vi "Misc.vi"   [LabVIEW 2018]
uses:
  <vilib>/Rock Robotics/WPI/DriverStation/WPI_DriverStationRobotMode2.ctl
  <vilib>/Rock Robotics/Network Tables/NT Read Boolean.vi
  SubSystems/Drive Train/Drive Train Global.vi
  <vilib>/Rock Robotics/Network Tables/NT Read String.vi
  Robot Global Data.vi
  SubSystems/HAB Climber/HAB Climber Global.vi
  <vilib>/Rock Robotics/Network Tables/NT Write Boolean.vi
  SubSystems/Lift/Lift Global.vi
  SubSystems/Cargo Intake/Cargo Intake Global.vi
  SubSystems/Hatch Panel Intake/Hatch Panel Intake Global.vi
  <vilib>/Rock Robotics/Network Tables/NT Write Numeric Array.vi
  <vilib>/Rock Robotics/Network Tables/NT Write Number.vi
  SubSystems/Controllers/Driver Controller/Driver Controller Global.vi
  SubSystems/Controllers/Manipulator Controlller/Manipulator Controller Global.vi
types:
  T1 = typedef "WPI_DriverStationRobotMode2.ctl" = enum16{"Autonomous Disabled", "Autonomous Enabled", "Teleop Disabled", "Teleop Enabled", "Disconnected", "Finish", "Test Disabled", "Test Enabled", "Emergency Stopped"}
  T2 = typedef "WPI_CompressorDevRef.ctl" = cluster{"DevStatus":errorcluster, "Pneumatics Control Module":u8}
  T3 = cluster{"FrontLeft":dbl, "FrontRight":dbl, "BackLeft":dbl, "BackRight":dbl}
  T4 = cluster{"Rollover":dbl, "Yaw":dbl, "Cont Yaw":dbl}
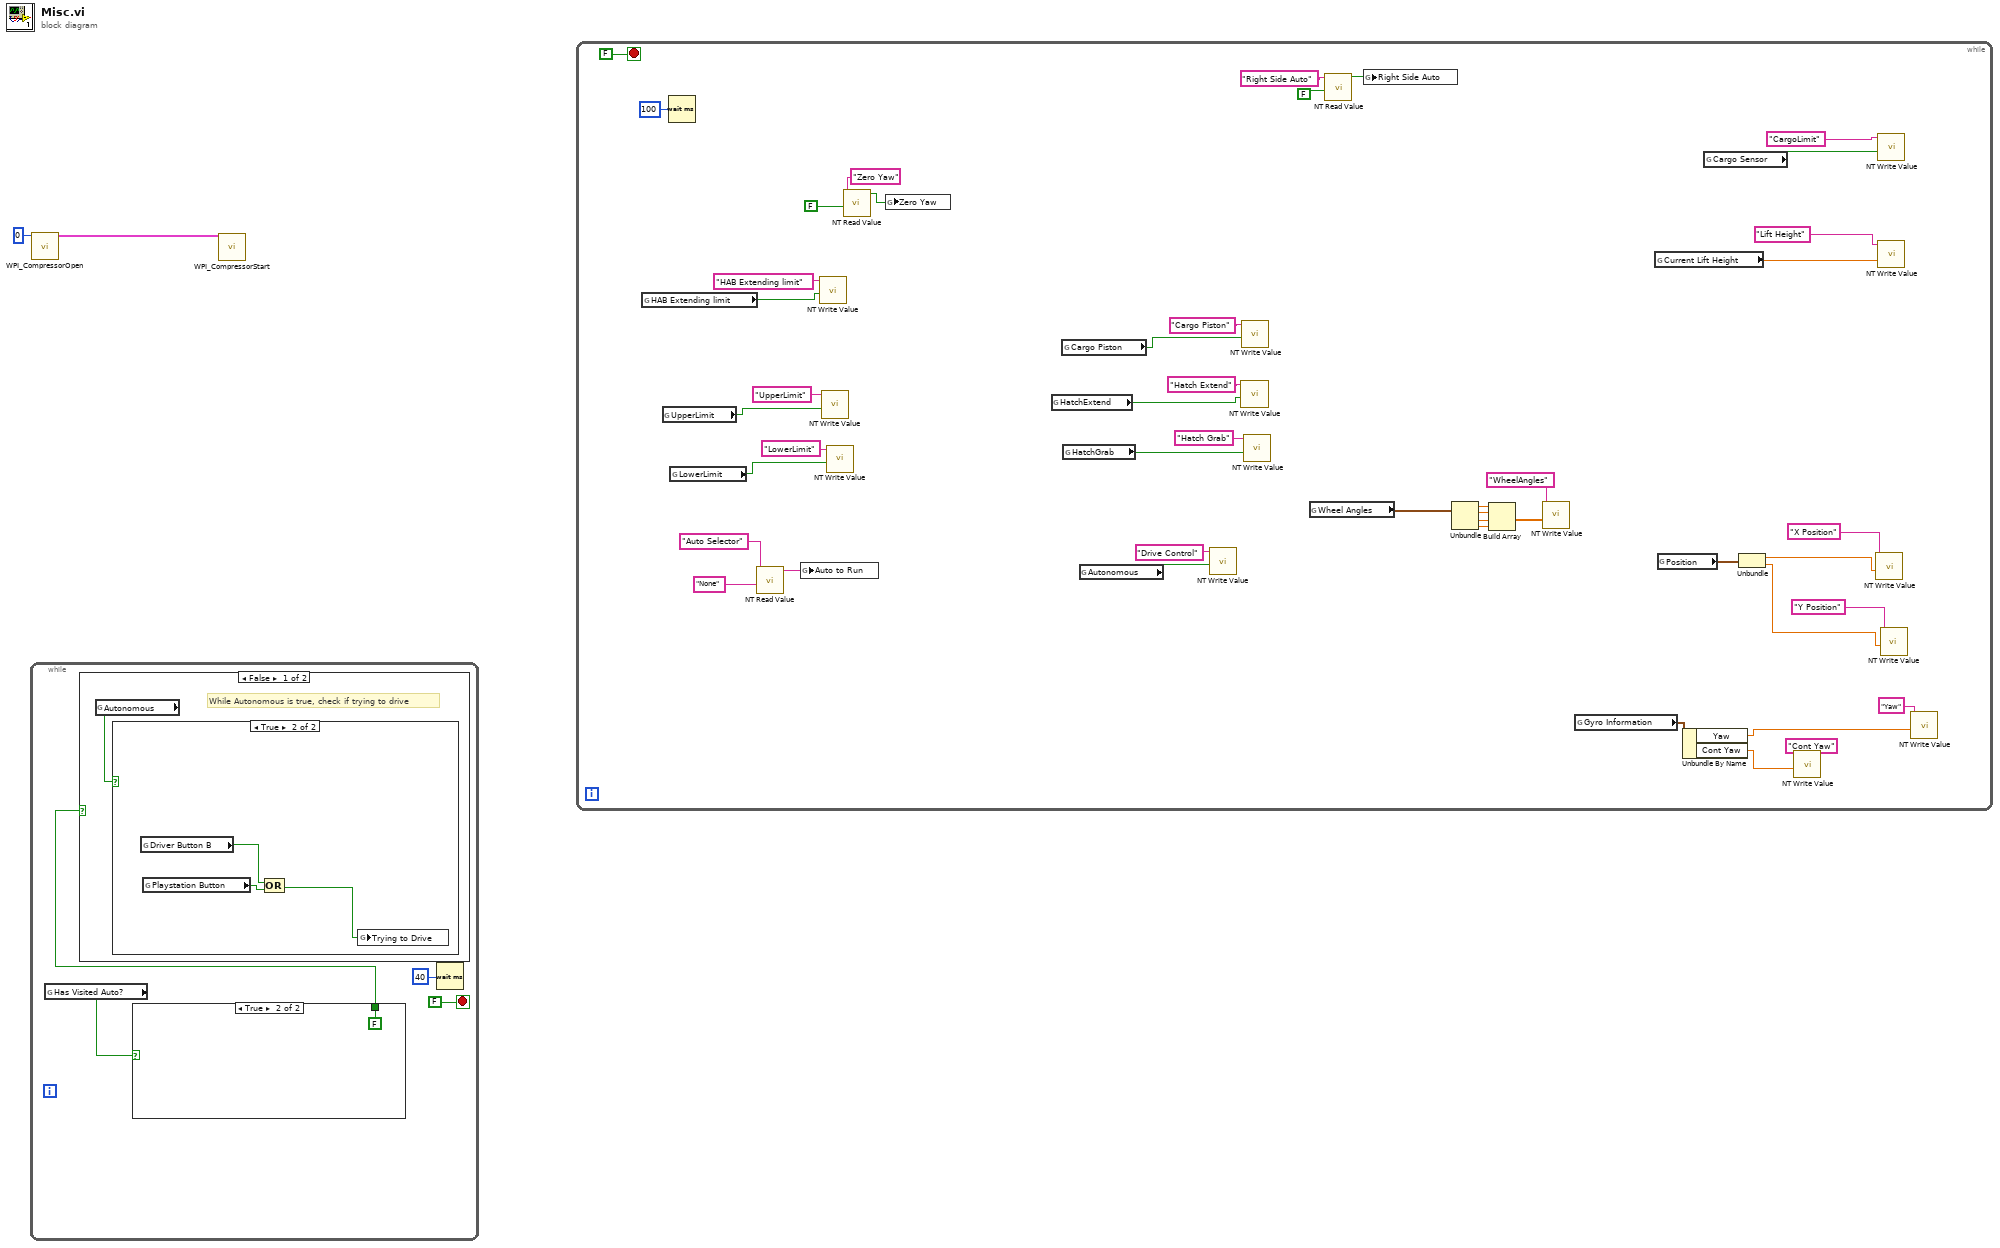
[diagram p0: block diagram]
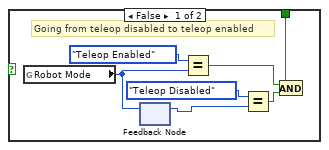
[diagram p2: hidden frame]
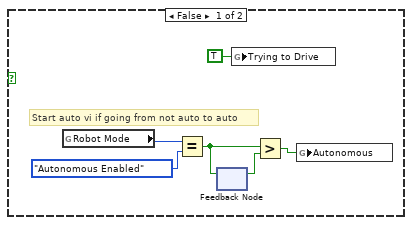
[diagram p3: hidden frame]
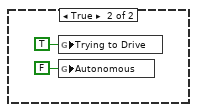
[diagram p4: hidden frame]
diagram:
  n1 = while {
    stop <- FALSE stop-if-true
    n2 = global read "Robot Global Data.vi" "Has Visited Auto?"() -> (w3:bool)
    n3 = case shown="True" w3 {
      tunnel: [w7 FALSE] -> w4
      frame False {
        # "Going from teleop disabled to teleop enabled"
        n4 = global read "Robot Global Data.vi" "Robot Mode"() -> (w13:T1)
        n5 = feedback #1() -> (w10:T1)  [unwired: 1 in]
        n6 = feedback-in #1(w13) -> ()
        n7 = Equal?(x=WPI_DriverStationRobotMode2."Teleop Enabled" ("y"), y=w13) -> (x = y?=w8:bool)
        n8 = Equal?(x=WPI_DriverStationRobotMode2."Teleop Disabled" ("y"), y=w10) -> (x = y?=w9:bool)
        n9 = And(x=w8, y=w9) -> (x .and. y?=w7:bool)
      }
      frame True {
      }
    }
    n10 = case shown="False" w4 {
      frame False {
        # "While Autonomous is true, check if trying to drive"
        n11 = global read "Robot Global Data.vi" "Autonomous"() -> (w15:bool)
        n12 = case shown="True" w15 {
          frame False {
            # "Start auto vi if going from not auto to auto"
            n13 = global read "Robot Global Data.vi" "Robot Mode"() -> (w17:T1)
            n14 = Equal?(x=w17, y=WPI_DriverStationRobotMode2."Autonomous Enabled") -> (x = y?=w18:bool)
            n15 = feedback #2() -> (w19:bool)  [unwired: 1 in]
            n16 = feedback-in #2(w18) -> ()
            n17 = global write "Robot Global Data.vi" "Trying to Drive"(TRUE ("Trying to Drive")) -> ()
            n18 = Greater?(x=w18, y=w19) -> (0:w20:bool)
            n19 = global write "Robot Global Data.vi" "Autonomous"(w20) -> ()
          }
          frame True {
            n20 = global read "Driver Controller Global.vi" "Driver Button B"() -> (w23:bool)
            n21 = global read "Manipulator Controller Global.vi" "Playstation Button"() -> (w22:bool)
            n22 = Compound Arithmetic op=OR(w23, w22) -> (w24:bool)
            n23 = global write "Robot Global Data.vi" "Trying to Drive"(w24) -> ()
          }
        }
      }
      frame True {
        n24 = global write "Robot Global Data.vi" "Trying to Drive"(TRUE ("Trying to Drive")) -> ()
        n25 = global write "Robot Global Data.vi" "Autonomous"(FALSE ("Autonomous")) -> ()
      }
    }
    n26 = Wait (ms)(milliseconds to wait=u32 40) -> ()  [unwired: 1 out]
  }
  n27 = call <vilib>:"WPI_CompressorOpen.vi"("Pneumatics Control Module (0)"=u8 0) -> ("CompressorDevRef"=w1:T2)  [unwired: 13 in, 1 out]
  n28 = call <vilib>:"WPI_CompressorStart.vi"("CompressorDevRef"=w1) -> ()  [unwired: 9 in, 2 out]
  n29 = while {
    stop <- FALSE stop-if-true
    n30 = global read "HAB Climber Global.vi" "HAB Extending limit"() -> (w65:bool)
    n31 = global read "Lift Global.vi" "UpperLimit"() -> (w64:bool)
    n32 = Wait (ms)(milliseconds to wait=u32 100) -> ()  [unwired: 1 out]
    n33 = global read "Lift Global.vi" "LowerLimit"() -> (w63:bool)
    n34 = call-poly <vilib>:"NT Read Value.vi"("Default Value"="None", "Name"="Auto Selector") -> ("String"=w46:string)  [unwired: 8 in, 1 out]
    n35 = global write "Robot Global Data.vi" "Auto to Run"(w46) -> ()
    n36 = call-poly <vilib>:"NT Write Value.vi"("Boolean"=w65, "Name"="HAB Extending limit") -> ()  [unwired: 9 in, 1 out]
    n37 = call-poly <vilib>:"NT Write Value.vi"("Boolean"=w64, "Name"="UpperLimit") -> ()  [unwired: 9 in, 1 out]
    n38 = call-poly <vilib>:"NT Write Value.vi"("Boolean"=w63, "Name"="LowerLimit") -> ()  [unwired: 9 in, 1 out]
    n39 = call-poly <vilib>:"NT Read Value.vi"("Default Value"=FALSE, "Name"="Zero Yaw") -> ("Boolean"=w69:bool)  [unwired: 8 in, 1 out]
    n40 = global write "Drive Train Global.vi" "Zero Yaw"(w69) -> ()
    n41 = global read "Hatch Panel Intake Global.vi" "HatchExtend"() -> (w57:bool)
    n42 = global read "Cargo Intake Global.vi" "Cargo Piston"() -> (w58:bool)
    n43 = global read "Hatch Panel Intake Global.vi" "HatchGrab"() -> (w56:bool)
    n44 = global read "Robot Global Data.vi" "Autonomous"() -> (w27:bool)
    n45 = call-poly <vilib>:"NT Write Value.vi"("Boolean"=w27, "Name"="Drive Control") -> ()  [unwired: 9 in, 1 out]
    n46 = call-poly <vilib>:"NT Write Value.vi"("Boolean"=w57, "Name"="Hatch Extend") -> ()  [unwired: 9 in, 1 out]
    n47 = call-poly <vilib>:"NT Write Value.vi"("Boolean"=w58, "Name"="Cargo Piston") -> ()  [unwired: 9 in, 1 out]
    n48 = call-poly <vilib>:"NT Write Value.vi"("Boolean"=w56, "Name"="Hatch Grab") -> ()  [unwired: 9 in, 1 out]
    n49 = global read "Drive Train Global.vi" "Wheel Angles"() -> (w55:T3)
    n50 = call-poly <vilib>:"NT Read Value.vi"("Default Value"=FALSE, "Name"="Right Side Auto") -> ("Boolean"=w32:bool)  [unwired: 8 in, 1 out]
    n51 = global write "Robot Global Data.vi" "Right Side Auto"(w32) -> ()
    n52 = Unbundle(w55) -> ("FrontLeft"=w51:dbl, "FrontRight"=w52:dbl, "BackLeft"=w53:dbl, "BackRight"=w54:dbl)
    n53 = Build Array(w51, w52, w53, w54) -> (w50:dbl[])
    n54 = call-poly <vilib>:"NT Write Value.vi"("Numeric Array"=w50, "Name"="WheelAngles") -> ()  [unwired: 9 in, 1 out]
    n55 = global read "Drive Train Global.vi" "Gyro Information"() -> (w40:T4)
    n56 = global read "Lift Global.vi" "Current Lift Height"() -> (w43:dbl)
    n57 = global read "Drive Train Global.vi" "Position"() -> (w38:cluster{"X":dbl, "Y":dbl})
    n58 = Unbundle By Name(w40) -> ("Yaw"=w30:dbl, "Cont Yaw"=w29:dbl)
    n59 = global read "Cargo Intake Global.vi" "Cargo Sensor"() -> (w45:bool)
    n60 = Unbundle(w38) -> ("X"=w36:dbl, "Y"=w34:dbl)
    n61 = call-poly <vilib>:"NT Write Value.vi"("Numeric"=w29, "Name"="Cont Yaw") -> ()  [unwired: 9 in, 1 out]
    n62 = call-poly <vilib>:"NT Write Value.vi"("Numeric"=w36, "Name"="X Position") -> ()  [unwired: 9 in, 1 out]
    n63 = call-poly <vilib>:"NT Write Value.vi"("Boolean"=w45, "Name"="CargoLimit") -> ()  [unwired: 9 in, 1 out]
    n64 = call-poly <vilib>:"NT Write Value.vi"("Numeric"=w43, "Name"="Lift Height") -> ()  [unwired: 9 in, 1 out]
    n65 = call-poly <vilib>:"NT Write Value.vi"("Numeric"=w34, "Name"="Y Position") -> ()  [unwired: 9 in, 1 out]
    n66 = call-poly <vilib>:"NT Write Value.vi"("Numeric"=w30, "Name"="Yaw") -> ()  [unwired: 9 in, 1 out]
  }
